vi "Query Output State.vi"(8 "error in (no error)":errorcluster, 9 "output state (Constant Voltage)":i32(ring) items=["Constant Voltage"=0, "Constant Current"=1, "Unregulated"=4, "Over Voltage"=2, "Over Current"=3], 10 "channel name (\"CHANNEL1\")":string="CHANNEL1", 11 "CS++DCPwr in":refnum<class "CS++DCPwr.lvclass">) -> (0 "error out":errorcluster, 2 "in state":bool, 3 "CS++DCPwr out":refnum<class "CS++DCPwr.lvclass">)   [LabVIEW 2013, in "CS++DCPwr.lvlib" / "CS++DCPwr.lvclass"]
doc: "This VI returns whether the power supply is in a particular output state.\n\nA constant voltage condition occurs when the output voltage is equal to the value of the IviDCPwr>>Basic Operation>>Voltage Level property and the current is less than or equal to the value of the IviDCPwr>>Basic Operation>>Current Limit property.\n\nA constant current condition occurs when the output current is equal to the value of the IviDCPwr>>Basic Operation>>Current Limit property and the IviDCPwr>>Basic Operation>>Current Limit Behavior property is set to IVIDCPWR_VAL_CURRENT_REGULATE.\n\nAn unregulated condition occurs when the output voltage is less than the value of the IviDCPwr>>Basic Operation>>Voltage Level property and the current is less than the value of the IviDCPwr>>Basic Operation>>Current Limit property.\n\nAn over-voltage condition occurs when the output voltage is equal to or greater than the value of the IviDCPwr>>Basic Operation>>OVP Limit property and the IviDCPwr>>Basic Operation>>OVP Enabled property is set to TRUE.\n\nAn over-current condition occurs when the output current is equal to or greater than the value of the IviDCPwr>>Basic Operation>>Current Limit property and the IviDCPwr>>Basic Operation>>Current Limit Behavior property is set to IVIDCPWR_VAL_CURRENT_TRIP. \n\nWhen either an over-voltage condition or an over-current condition occurs, the power supply's output protection disables the output. If the power supply is in an over-voltage or over-current state, it does not produce power until the output protection is reset. The IviDCPwr Reset Output Protection VI resets the output protection. Once the output protection is reset, the power supply resumes generating a power signal."
uses:
  CS++DCPwr.lvclass
  Core/Classes/CS++ProcessVariables/ProcessVariable/PV.lvclass
  CS++DCPwr.lvclass/CS++DCPwr.ctl
  Core/Classes/CS++ProcessVariables/PVConnection/PVConnection.lvclass
  Core/Classes/CS++ProcessVariables/ProcessVariable/PV.lvclass/PV.ctl
  Core/Classes/CS++ProcessVariables/ProcessVariable/Write Data.vi
  Core/Classes/CS++ProcessVariables/ProcessVariable/Write Timestamp.vi
  Core/Classes/CS++ProcessVariables/ProcessVariable/Write Quality.vi
  Core/Classes/CS++ProcessVariables/ProcessVariable/Write status.vi
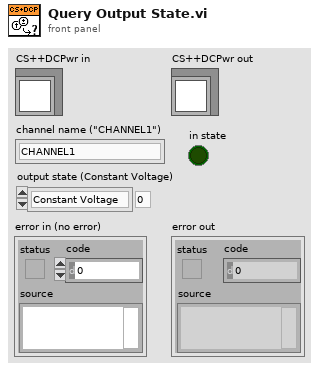
[diagram p1: front panel]
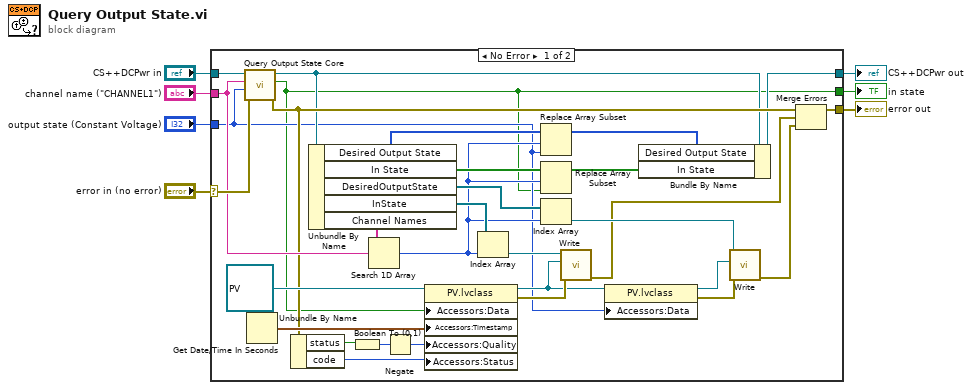
[diagram p0: block diagram]
diagram:
  n1 = case shown="No Error" "error in (no error)" {
    selector: "error in (no error)" -> [w37 w40]
    tunnel: [w29 w40] -> w6
    tunnel: [w20 w39] -> w4
    tunnel: "CS++DCPwr in" -> [w38 w39]
    tunnel: "channel name (\"CHANNEL1\")" -> [w32 _]
    tunnel: "output state (Constant Voltage)" -> [w11 _]
    tunnel: [w8 _] -> w1
    frame No Error {
      n2 = call-dynamic "Query Output State Core.vi"("error in (no error)"=w37, "output state (Constant Voltage)"=w11, "channel name (\"CHANNEL1\")"=w32, "CS++DCPwr in"=w38) -> ("error out"=w24:errorcluster, "in state"=w8:bool, "CS++DCPwr out"=w21:refnum<class "CS++DCPwr.lvclass">)  [unwired: 5 in]
      n3 = Get Date/Time In Seconds() -> (seconds since 1Jan1904=w36:timestamp)
      n4 = Unbundle By Name(w24) -> ("status"=w28:bool, "code"=w26:i32)
      n5 = Unbundle By Name(w21) -> ("Desired Output State"=w19:i32[], "In State"=w23:bool[], "DesiredOutputState"=w14:refnum<class "PVConnection.lvclass">[], "InState"=w31:refnum<class "PVConnection.lvclass">[], "Channel Names"=w33:string[])
      n6 = Boolean To (0,1)(Boolean=w28) -> (0, 1=w27:i16)
      n7 = Search 1D Array(1D array=w33, element=w32) -> (index of element=w13:i32)  [unwired: 1 in]
      n8 = Negate(x=w27) -> (-x=w25:i16)
      n9 = property class="PV.lvclass"(reference=refnum<class "PV.lvclass"> refnum ("PV"), "Accessors:Data"=w8, "Accessors:Timestamp"=w36, "Accessors:Quality"=w25, "Accessors:Status"=w26) -> (reference out=w12:refnum<class "PV.lvclass">, error out=w34:errorcluster)  [unwired: 1 in]
      n10 = Index Array(array=w31, index=w13) -> (element=w30:refnum<class "PVConnection.lvclass">)
      n11 = Replace Array Subset(array=w19, new element=w11, index=w13) -> (w18:i32[])
      n12 = Replace Array Subset(array=w23, new element=w8, index=w13) -> (w22:bool[])
      n13 = Index Array(array=w14, index=w13) -> (element=w17:refnum<class "PVConnection.lvclass">)
      n14 = call-dynamic "Write.vi"("error in (no error)"=w34, "PV"=w12, "PVConnection in"=w30) -> ("error out"=w10:errorcluster)  [unwired: 7 in, 1 out]
      n15 = property class="PV.lvclass"(reference=w12, "Accessors:Data"=w11) -> (reference out=w16:refnum<class "PV.lvclass">, error out=w15:errorcluster)  [unwired: 1 in]
      n16 = Bundle By Name(cluster=w21, "Desired Output State"=w18, "In State"=w22) -> (w20:refnum<class "CS++DCPwr.lvclass">)
      n17 = call-dynamic "Write.vi"("error in (no error)"=w15, "PV"=w16, "PVConnection in"=w17) -> ("error out"=w9:errorcluster)  [unwired: 7 in, 1 out]
      n18 = Merge Errors(w24, w10, w9) -> (w29:errorcluster)
    }
    frame Error {
    }
  }
  "error out" <- w6
  "CS++DCPwr out" <- w4
  "in state" <- w1
